vi "Load Config.vi"(6 "Constants":refnum<class "Sequence Constants.lvclass">, 8 "error in (no error)":refnum<class "MultiErrors.lvclass">, 10 "Config Element":refnum<class "Config Element.lvclass">, 11 "Command Config in":refnum<class "Command Config.lvclass">) -> (0 "error out":refnum<class "MultiErrors.lvclass">, 3 "Command Config out":refnum<class "Command Config.lvclass">)   [LabVIEW 2020, in "VolatusSeqConfig.lvlib" / "Command Config.lvclass"]
uses:
  Command Config.lvclass
  VolatusErrorUtilities/MultiErrors/MultiErrors.lvclass
  lv-cdm/CDM-Config/Config Element/Config Element.lvclass
  Command Config.lvclass/Command Config.ctl
  Sequence Constants/Sequence Constants.lvclass
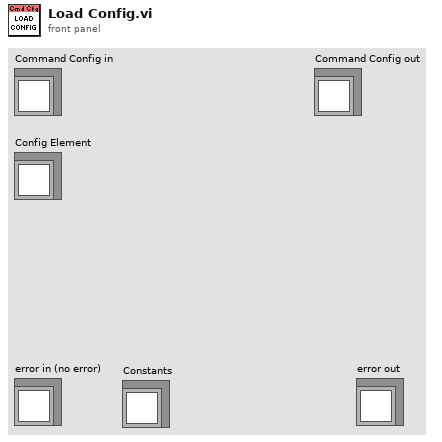
[diagram p1: front panel]
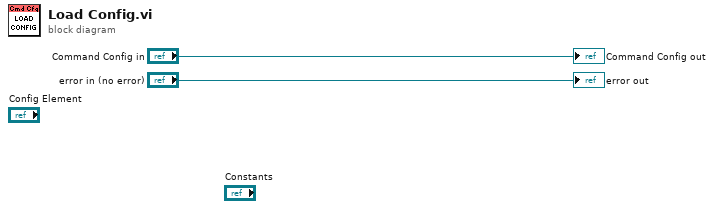
[diagram p0: block diagram]
diagram:
  "error out" <- "error in (no error)"
  "Command Config out" <- "Command Config in"
